vi "Configure Output Timer.vi"(5 "Duration (1 s)":i32=1, 6 "Current Level (0 A)":dbl, 7 "Voltage Level (0 V)":dbl, 8 "error in (no error)":errorcluster, 9 "Timer Number (1)":i32=1, 10 "Channel (0: +6V Channel)":i32(ring) caption="Channel (0: +6V)" items=["+6V Channel", "+25V Channel", "-25V Channel"], 11 "VISA resource name":refnum<visa-resource-name>) -> (0 "error out":errorcluster, 3 "VISA resource name out":refnum<visa-resource-name>)   [LabVIEW 2020, in "RIGOL DP1000 Series.lvlib"]
doc: "Configures the output timer function."
uses:
  <instrlib>/RIGOL DP1000 Series/RIGOL DP1000 Series.lvlib
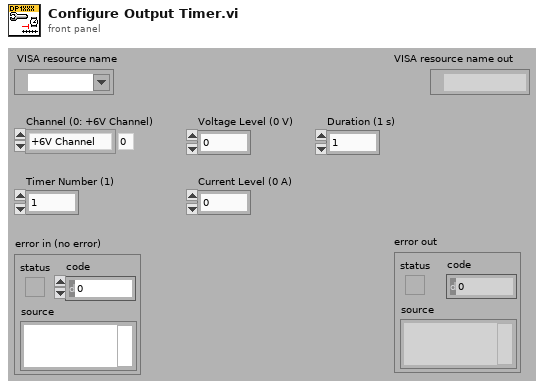
[diagram p1: front panel]
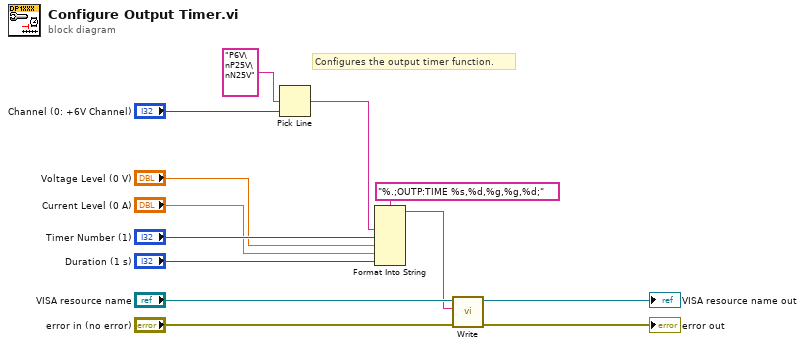
[diagram p0: block diagram]
diagram:
  # "Configures the output timer function."
  n1 = Pick Line(multi-line string="P6V\nP25V\nN25V", line index="Channel (0: +6V Channel)") -> (output string=w10:string)  [unwired: 1 out]
  n2 = Format Into String(format string="%.;OUTP:TIME %s,%d,%g,%g,%d;", w10, "Timer Number (1)", "Voltage Level (0 V)", "Current Level (0 A)", "Duration (1 s)") -> (resulting string=w1:string)  [unwired: 2 in, 1 out]
  n3 = call <instrlib>:"Write.vi"("error in (no error)"="error in (no error)", "Write Buffer (\"\")"=w1, "VISA resource name"="VISA resource name") -> ("error out"=→"error out":errorcluster, "VISA resource name out"=→"VISA resource name out":refnum<visa-resource-name>)  [unwired: 7 in]
